vi "Call.vi"(0 "Arguments":cluster{string, dbl}[](array[cluster]), 1 "Function or Method Name":string, 2 "Path to Python Module (.py file)":path) -> ()   [LabVIEW 2015]
panel:
  out "standard error":string
  out "standard output":string
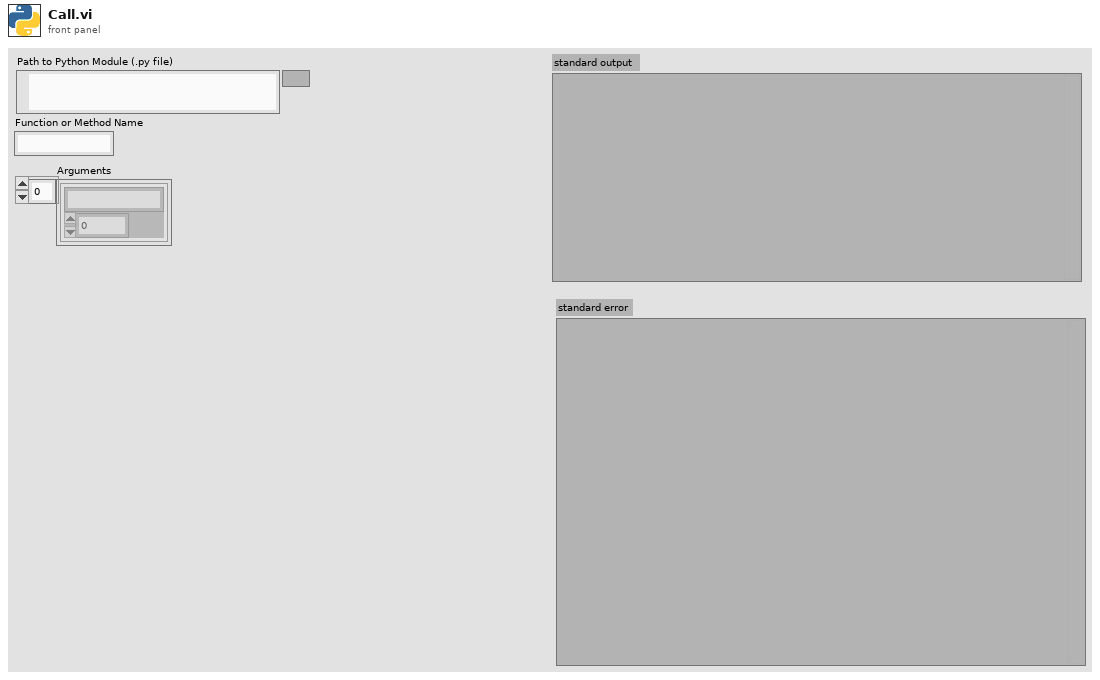
[diagram p1: front panel]
types:
  T1 = cluster{"module":string, "function":string, "arguments":cluster{string, dbl}[]}
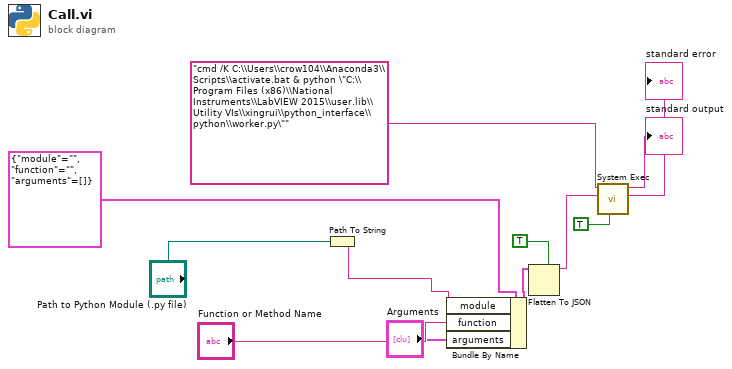
[diagram p0: block diagram]
diagram:
  n1 = Path To String(path="Path to Python Module (.py file)") -> (string=w5:string)
  n2 = Bundle By Name(cluster=T1 {"module"="", "function"="", "arguments"=[]}, "module"=w5, "function"="Function or Method Name", "arguments"="Arguments") -> (w4:T1)
  n3 = Flatten To JSON(enable LabVIEW extensions? (T)=TRUE, anything=w4) -> (JSON string=w8:string)  [unwired: 1 in, 1 out]
  n4 = call <vilib>:"System Exec.vi"("run minimized? (F)"=TRUE, "standard input"=w8, "command line"="cmd /K C:\\Users\\crow104\\Anaconda3\\Scripts\\activate.bat & python \"C:\\Program Files (x86)\\National Instruments\\LabVIEW 2015\\user.lib\\Utility VIs\\xingrui\\python_interface\\python\\worker.py\"") -> ("standard error"=→"standard error":string, "standard output"=→"standard output":string)  [unwired: 5 in, 2 out]
